vi "GPS.vi"() -> ()   [LabVIEW 2014]
panel:
  out "GPS Lat, Long, Dev":dbl[](array[numeric]) format="%#_8g"
  in  "stop":bool
  in  "GPS COM Port":refnum<visa-resource-name>
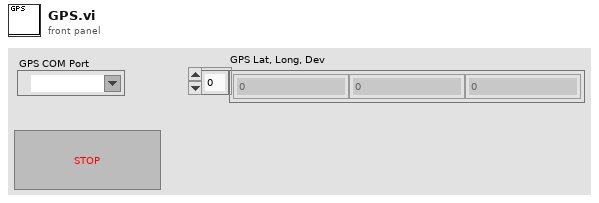
[diagram p1: front panel]
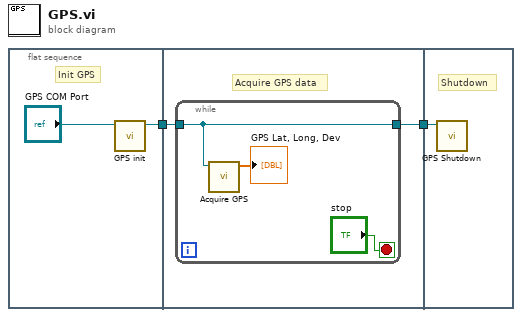
[diagram p0: block diagram]
diagram:
  n1 = flat-sequence {
    tunnel: [w3] -> w2
    tunnel: w2 -> [w6]
    tunnel: [w5] -> w1
    tunnel: w1 -> [w10]
    frame #0 {
      # "Init GPS"
      n2 = call "GPS init.vi"("VISA resource name in"="GPS COM Port") -> ("VISA resource name out"=w3:refnum<visa-resource-name>)  [unwired: 10 in]
    }
    frame #1 {
      # "Acquire GPS data"
      n3 = while {
        tunnel: w6 -> [w8]
        tunnel: [w8] -> w5
        stop <- "stop" stop-if-true
        n4 = call "Acquire GPS.vi"("GPS COM Port"=w8) -> ("Lat, long, dev output"=→"GPS Lat, Long, Dev":dbl[])  [unwired: 10 in]
      }
    }
    frame #2 {
      # "Shutdown"
      n5 = call "GPS Shutdown.vi"("GPS COM port"=w10) -> ()  [unwired: 11 in]
    }
  }
